vi "Repair Linkage.vi"(10 "Status":refnum<vi>, 11 "WebView2 Updater in":refnum<class "WebView2 Updater.lvclass">) -> (0 "error out":errorcluster)   [LabVIEW 2020, in "WebView2 Updater.lvclass"]
uses:
  WebView2 Updater.lvclass
  WebView2 Updater.lvclass/WebView2 Updater.ctl
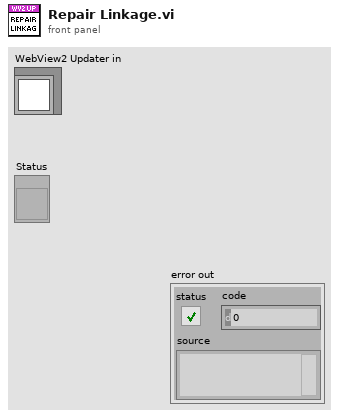
[diagram p1: front panel]
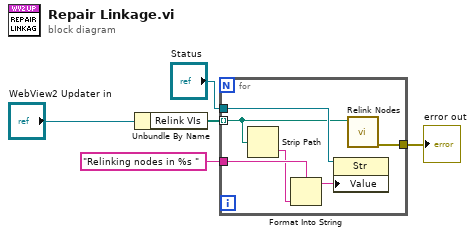
[diagram p0: block diagram]
diagram:
  n1 = Unbundle By Name("WebView2 Updater in") -> ("Relink VIs"=w1:path[])
  n2 = for {
    tunnel: "Relinking nodes in %s " ("format string") -> [w11]
    tunnel: [w9] -> w5
    tunnel: "Status" -> [w8]
    tunnel: w1 -> [w7] mode=indexing
    n3 = Strip Path(path=w7) -> (name=w6:string)  [unwired: 1 out]
    n4 = Format Into String(format string=w11, w6) -> (resulting string=w10:string)  [unwired: 2 in, 1 out]
    n5 = property class="Str"(reference=w8, "Value"=w10) -> ()  [unwired: 1 in, 2 out]
    n6 = call "Relink Nodes.vi"("Path"=w7) -> ("error out"=w9:errorcluster)  [unwired: 10 in]
  }
  "error out" <- w5
